vi "SVXMPL_Get Wav subset.vi"(4 "selection has changed":bool, 6 "block size":dbl=1024.0 format="%.2f", 8 "error in (no error)":errorcluster, 10 "number of samples":i32, 11 "waveform in":waveform(dbl)) -> (0 "error out":errorcluster, 2 "start":dbl format="%.2f", 3 "signal [V]":waveform(dbl))   [LabVIEW 2017]
uses:
  <vilib>/Waveform/WDTOps.llb/WDT Get Waveform Subset DBL (LV80).vi
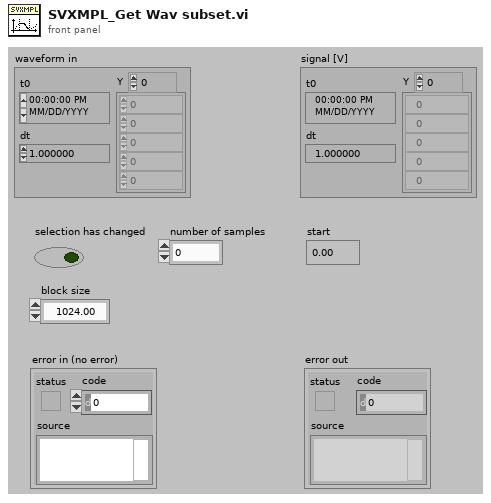
[diagram p1: front panel]
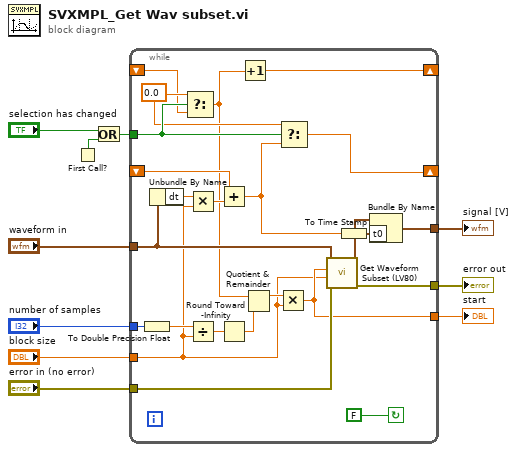
[diagram p0: block diagram]
diagram:
  n1 = First Call?() -> (First Call?: T/F=w2:bool)
  n2 = Or(x="selection has changed", y=w2) -> (x .or. y?=w3:bool)
  n3 = while {
    tunnel: w3 -> [w16]
    shift-left: _ -> [w14]
    shift-right: [w13] -> _
    tunnel: [w17] -> w4
    shift-left: _ -> [w27]
    shift-right: [w26] -> _
    tunnel: "waveform in" -> [w23]
    tunnel: "block size" -> [w18]
    tunnel: [w21] -> w7
    tunnel: [w32] -> w8
    tunnel: "number of samples" -> [w33]
    tunnel: "error in (no error)" -> [w34]
    stop <- FALSE continue-if-true
    w15 = 0.0 ("t")
    n4 = To Double Precision Float(number=w33) -> (double precision float=w20:dbl)
    n5 = Unbundle By Name(w23) -> ("dt"=w29:dbl)
    n6 = Select(t=w15, s=w16, f=w14) -> (s? t:f=w12:dbl)
    n7 = Multiply(x=w29, y=w18) -> (x*y=w28:dbl)
    n8 = Divide(x=w20, y=w18) -> (x/y=w31:dbl)
    n9 = Add(x=w27, y=w28) -> (x+y=w25:dbl)
    n10 = Round Toward -Infinity(1:w31) -> (0:w24:dbl)
    n11 = Increment(x=w12) -> (x+1=w13:dbl)
    n12 = Quotient & Remainder(x=w12, y=w24) -> (x-y*floor(x/y)=w19:dbl)  [unwired: 1 out]
    n13 = Multiply(x=w19, y=w18) -> (x*y=w32:dbl)
    n14 = Select(t=w15, s=w16, f=w25) -> (s? t:f=w26:dbl)
    n15 = call-poly <vilib>:"Get Waveform Subset (LV80).vi"("error in (no error)"=w34, "duration"=w18, "start samples/time"=w32, "waveform in"=w23) -> ("error out"=w17:errorcluster, "waveform out"=w22:waveform(dbl))  [unwired: 2 in, 2 out]
    n16 = To Time Stamp(1:w25) -> (0:w11:timestamp)
    n17 = Bundle By Name(cluster=w22, "t0"=w11) -> (w21:waveform(dbl))
  }
  "start" <- w8
  "error out" <- w4
  "signal [V]" <- w7
